vi "voltage_referenced_motor_command.vi"(10 "vsup_volts":sgl, 11 "des_volts":sgl) -> (3 "motor_cmd":sgl)   [LabVIEW 2013]
panel:
  in  "Min VBatt":sgl=4.0
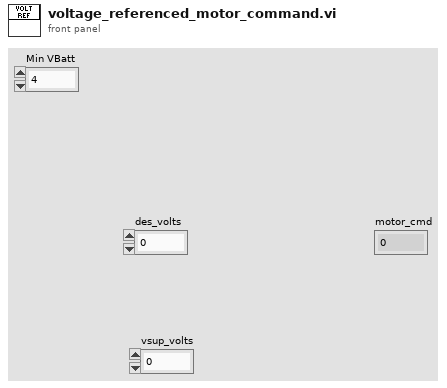
[diagram p1: front panel]
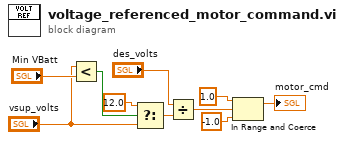
[diagram p0: block diagram]
diagram:
  n1 = Less?(x="vsup_volts", y="Min VBatt") -> (x < y?=w3:bool)
  n2 = Select(t=sgl 12.0, s=w3, f="vsup_volts") -> (s? t:f=w2:sgl)
  n3 = Divide(x="des_volts", y=w2) -> (x/y=w5:sgl)
  n4 = In Range and Coerce(upper limit=sgl 1.0, x=w5, lower limit=sgl -1.0) -> (coerced(x)=→"motor_cmd":sgl)  [unwired: 1 out]
